vi "Box.vi"(8 "error in (no error)":errorcluster, 11 "Pizza in":refnum<class "Pizza.lvclass">) -> (0 "error out":errorcluster, 3 "Pizza out":refnum<class "Pizza.lvclass">)   [LabVIEW 2020, in "FactoryMethod.lvlib" / "PizzaFactoryMethod.lvlib" / "Pizza.lvclass"]
uses:
  Pizza.lvclass
  Pizza.lvclass/Pizza.ctl
  Support/Class/ConsoleOutput.lvclass
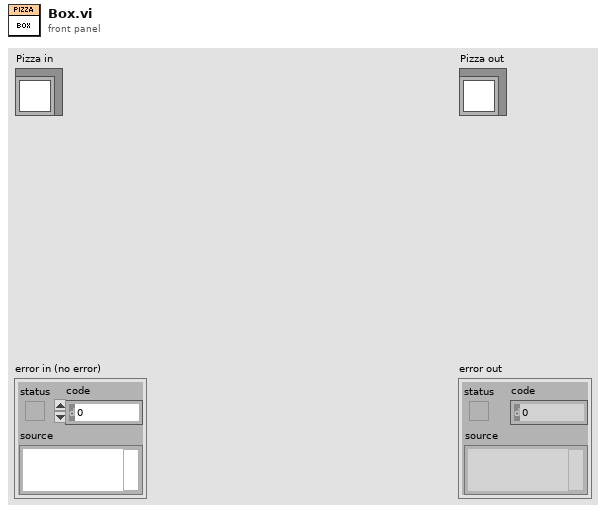
[diagram p1: front panel]
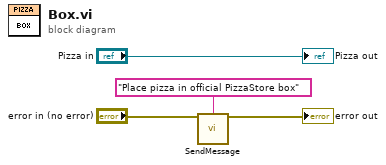
[diagram p0: block diagram]
diagram:
  n1 = call "SendMessage.vi"("Message"="Place pizza in official PizzaStore box", "error in (no error)"="error in (no error)") -> ("error out"=→"error out":errorcluster)  [unwired: 13 in]
  "Pizza out" <- "Pizza in"
